vi "UtilityLib.zip.vi"(0 "zipFilePath":path, 1 "sourcePath":path, 2 "foldersToExclude":string[](array[string]), 3 "recursionType":T1(ring), 5 "error in (no error)":errorcluster, 7 "previewOnly":bool) -> (14 "dup zipFilePath":path, 15 "zippedFiles":path[](array[path]), 19 "error out":errorcluster)   [LabVIEW 2014, in "UtilityLib.lvlib"]
doc: "Zips a file, directory or recursive directory. This deletes and rewrites the file if it already exists. You cannot append data to a zip file."
uses:
  UtilityLib.lvlib
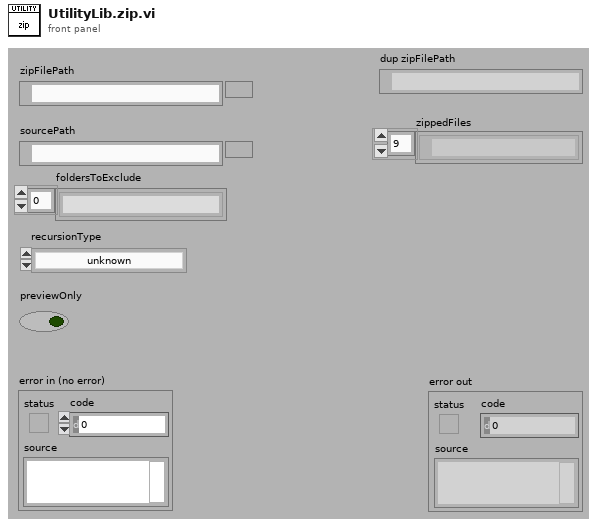
[diagram p1: front panel]
types:
  T1 = enum16{"unknown", "recursive", "specifiedFolderOnly", "singleFile"}
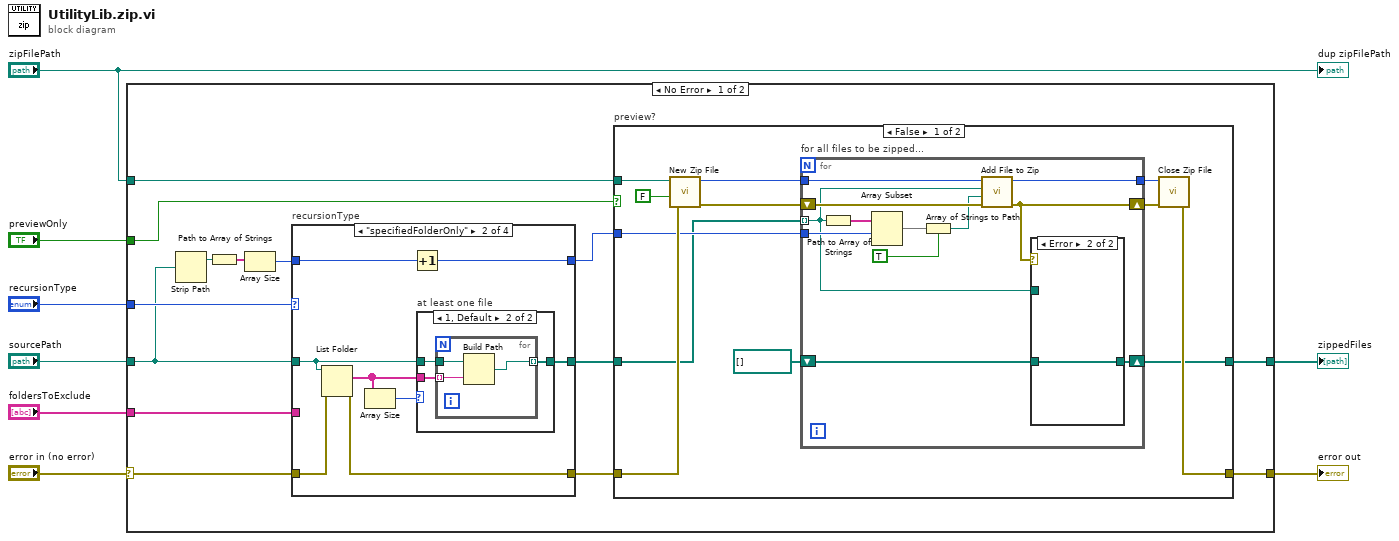
[diagram p0: block diagram]
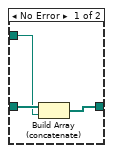
[diagram p2: hidden frame]
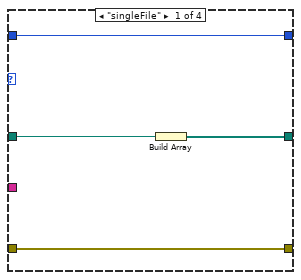
[diagram p4: hidden frame]
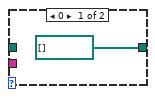
[diagram p5: hidden frame]
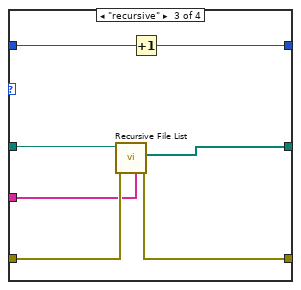
[diagram p6: hidden frame]
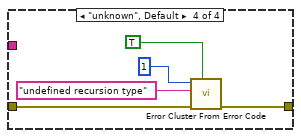
[diagram p7: hidden frame]
diagram:
  n1 = case shown="No Error" "error in (no error)" {
    selector: "error in (no error)" -> [w11 w84]
    tunnel: "zipFilePath" -> [w22 _]
    tunnel: "foldersToExclude" -> [w21 _]
    tunnel: "recursionType" -> [w20 _]
    tunnel: [w17 w84] -> w6
    tunnel: [w16 _] -> w5
    tunnel: "sourcePath" -> [w13 _]
    tunnel: "previewOnly" -> [w12 _]
    frame No Error {
      n2 = Strip Path(path=w13) -> (stripped path=w14:path)  [unwired: 1 out]
      n3 = Path to Array of Strings(0:w14) -> (2:w15:string[])  [unwired: 1 out]
      n4 = Array Size(array=w15) -> (size(s)=w10:i32)
      n5 = case "recursionType" shown="\"specifiedFolderOnly\"" w20 {
        tunnel: w13 -> [w55 w62 w78 _]
        tunnel: w11 -> [w56 w61 w77 w83]
        tunnel: [w56 w60 w76 w82] -> w19
        tunnel: w21 -> [_ _ w75 _]
        tunnel: [w54 w59 w74 _] -> w18
        tunnel: w10 -> [w53 w58 w73 _]
        tunnel: [w53 w57 w72 _] -> w9
        frame "singleFile" {
          n6 = Build Array(w55) -> (w54:path[])
        }
        frame "specifiedFolderOnly" {
          n7 = List Folder(path=w62, error in=w61) -> (filenames=w63:string[], error out=w60:errorcluster)  [unwired: 2 in, 2 out]
          n8 = Array Size(array=w63) -> (size(s)=w64:i32)
          n9 = Increment(x=w58) -> (x+1=w57:i32)
          n10 = case "at least one file" shown="1, Default" w64 {
            tunnel: w63 -> [_ w68]
            tunnel: w62 -> [_ w67]
            tunnel: [path[] [] w66] -> w59
            frame 0 {
            }
            frame 1, Default {
              n11 = for {
                tunnel: w68 -> [w70] mode=indexing
                tunnel: w67 -> [w71]
                tunnel: [w69] -> w66 mode=indexing
                n12 = Build Path(base path=w71, name or relative path=w70) -> (appended path=w69:path)
              }
            }
          }
        }
        frame "recursive" {
          n13 = call <vilib>:"Recursive File List.vi"("Folders to Exclude"=w75, "error in (no error)"=w77, "Folder Path"=w78) -> ("error out"=w76:errorcluster, "All Files in Dir"=w74:path[])  [unwired: 4 in, 3 out]
          n14 = Increment(x=w73) -> (x+1=w72:i32)
        }
        frame "unknown", Default {
          n15 = call <vilib>:"Error Cluster From Error Code.vi"("show call chain? (False)"=TRUE, "error in (no error)"=w83, "error message (\"\")"="undefined recursion type" ("error message (\"\")"), "error code (0)"=1) -> ("error out"=w82:errorcluster)  [unwired: 5 in]
        }
      }
      n16 = case "preview?" shown="False" w12 {
        tunnel: w22 -> [w34 _]
        tunnel: w19 -> [w32 w52]
        tunnel: w18 -> [w25 w51]
        tunnel: [w27 w52] -> w17
        tunnel: [w23 w51] -> w16
        tunnel: w9 -> [w26 _]
        frame False {
          n17 = call <vilib>:"New Zip File.vi"("error in (no error)"=w32, "confirm overwrite? (F)"=FALSE, "target"=w34) -> ("error out"=w30:errorcluster, "zip file out"=w31:i64)  [unwired: 2 in, 1 out]
          n18 = for "for all files to be zipped..." {
            tunnel: w31 -> [w46]
            tunnel: w25 -> [w36] mode=indexing
            shift-right: [w38] -> w28
            shift-left: w30 -> [w45]
            tunnel: [w44] -> w29
            tunnel: w26 -> [w42]
            shift-right: [w35] -> w23
            shift-left: path[] [] -> [w37]
            n19 = Path to Array of Strings(0:w36) -> (2:w43:string[])  [unwired: 1 out]
            n20 = Array Subset(array=w43, index=w42) -> (w40:string[])  [unwired: 1 in]
            n21 = Array of Strings to Path(0:w40, 1:TRUE ("relative")) -> (2:w39:path)
            n22 = call <vilib>:"Add File to Zip.vi"("error in (no error)"=w45, "destination path in zip"=w39, "source file path"=w36, "zip file in"=w46) -> ("error out"=w38:errorcluster, "zip file out"=w44:i64)  [unwired: 6 in]
            n23 = case shown="Error" w38 {
              tunnel: w37 -> [w49 w50]
              tunnel: w36 -> [w48 _]
              tunnel: [w47 w50] -> w35
              frame No Error {
                n24 = Build Array (concatenate)(w49, w48) -> (w47:path[])
              }
              frame Error {
              }
            }
          }
          n25 = call <vilib>:"Close Zip File.vi"("error in (no error)"=w28, "zip file in"=w29) -> ("error out"=w27:errorcluster)  [unwired: 5 in]
        }
        frame True {
        }
      }
    }
    frame Error {
    }
  }
  "error out" <- w6
  "zippedFiles" <- w5
  "dup zipFilePath" <- "zipFilePath"
